vi "c Spark Get Parameter Type.vi"(8 "error in (no error)":errorcluster, 10 "paramID":T1 items=["   c_Spark_kCANID "=0, "    c_Spark_kInputMode "=1, "    c_Spark_kMotorType "=2, "    c_Spark_kCommutationAdvance "=3, "    c_Spark_kControlType "=5, "    c_Spark_kIdleMode "=6, "    c_Spark_kInputDeadband "=7, "    c_Spark_kClosedLoopControlSensor "=9, "    c_Spark_kPolePairs "=10, "    c_Spark_kCurrentChop "=11, "    c_Spark_kCurrentChopCycles "=12, "    c_Spark_kP_0 "=13, "    c_Spark_kI_0 "=14, "    c_Spark_kD_0 "=15, "    c_Spark_kV_0 "=16, "    c_Spark_kIZone_0 "=17, "    c_Spark_kDFilter_0 "=18, "    c_Spark_kOutputMin_0 "=19, "    c_Spark_kOutputMax_0 "=20, "    c_Spark_kP_1 "=21, "    c_Spark_kI_1 "=22, "    c_Spark_kD_1 "=23, "    c_Spark_kV_1 "=24, "    c_Spark_kIZone_1 "=25, "    c_Spark_kDFilter_1 "=26, "    c_Spark_kOutputMin_1 "=27, "    c_Spark_kOutputMax_1 "=28, "    c_Spark_kP_2 "=29, "    c_Spark_kI_2 "=30, "    c_Spark_kD_2 "=31, "    c_Spark_kV_2 "=32, "    c_Spark_kIZone_2 "=33, "    c_Spark_kDFilter_2 "=34, "    c_Spark_kOutputMin_2 "=35, "    c_Spark_kOutputMax_2 "=36, "    c_Spark_kP_3 "=37, "    c_Spark_kI_3 "=38, "    c_Spark_kD_3 "=39, "    c_Spark_kV_3 "=40, "    c_Spark_kIZone_3 "=41, "    c_Spark_kDFilter_3 "=42, "    c_Spark_kOutputMin_3 "=43, "    c_Spark_kOutputMax_3 "=44, "    c_Spark_kInverted "=45, "    c_Spark_kLimitSwitchFwdPolarity "=50, "    c_Spark_kLimitSwitchRevPolarity "=51, "    c_Spark_kHardLimitFwdEn "=52, "    c_Spark_kHardLimitRevEn "=53, "    c_Spark_kSoftLimitFwdEn "=54, "    c_Spark_kSoftLimitRevEn "=55, "    c_Spark_kOpenLoopRampRate "=56, "    c_Spark_kLegacyFollowerID "=57, "    c_Spark_kLegacyFollowerConfig "=58, "    c_Spark_kSmartCurrentStallLimit "=59, "    c_Spark_kSmartCurrentFreeLimit "=60, "    c_Spark_kSmartCurrentConfig "=61, "    c_Spark_kSmartCurrentReserved "=62, "    c_Spark_kMotorKv "=63, "    c_Spark_kEncoderCountsPerRev "=69, "    c_Spark_kEncoderAverageDepth "=70, "    c_Spark_kEncoderSampleDelta "=71, "    c_Spark_kEncoderInverted "=72, "    c_Spark_kVoltageCompensationMode "=74, "    c_Spark_kCompensatedNominalVoltage "=75, "    c_Spark_kIMaxAccum_0 "=96, "    c_Spark_kAllowedClosedLoopError_0 "=97, "    c_Spark_kIMaxAccum_1 "=100, "    c_Spark_kAllowedClosedLoopError_1 "=101, "    c_Spark_kIMaxAccum_2 "=104, "    c_Spark_kAllowedClosedLoopError_2 "=105, "    c_Spark_kIMaxAccum_3 "=108, "    c_Spark_kAllowedClosedLoopError_3 "=109, "    c_Spark_kClosedLoopRampRate "=114, "    c_Spark_kSoftLimitForward "=115, "    c_Spark_kSoftLimitReverse "=116, "    c_Spark_kAnalogAverageDepth "=121, "    c_Spark_kAnalogSensorMode "=122, "    c_Spark_kAnalogInverted "=123, "    c_Spark_kAnalogSampleDelta "=124, "    c_Spark_kCompatibilityPortConfig "=127, "    c_Spark_kAltEncoderCountsPerRev "=128, "    c_Spark_kAltEncoderAverageDepth "=129, "    c_Spark_kAltEncoderSampleDelta "=130, "    c_Spark_kAltEncoderInverted "=131, "    c_Spark_kNumParameters "=138, "    c_Spark_kDutyCycleInverted "=141, "    c_Spark_kDutyCycleAverageDepth "=143, "    c_Spark_kDutyCycleOffsetLegacy "=145, "    c_Spark_kDutyCycleRangeOffset "=146, "    c_Spark_kPositionPIDWrapEnable "=149, "    c_Spark_kDutyCycleSensorPrescaler "=153, "    c_Spark_kDutyCycleOffset "=154, "    c_Spark_kProductId "=155, "    c_Spark_kDeviceMajorVersion "=156, "    c_Spark_kDeviceMinorVersion "=157, "    c_Spark_kStatus0Period "=158, "    c_Spark_kStatus1Period "=159, "    c_Spark_kStatus2Period "=160, "    c_Spark_kStatus3Period "=161, "    c_Spark_kStatus4Period "=162, "    c_Spark_kStatus5Period "=163, "    c_Spark_kStatus6Period "=164, "    c_Spark_kStatus7Period "=165, "    c_Spark_kMAXMotionCruiseVelocity_0 "=166, "    c_Spark_kMAXMotionMaxAccel_0 "=167, "    c_Spark_kMAXMotionMaxJerk_0 "=168, "    c_Spark_kMAXMotionAllowedProfileError_0 "=169, "    c_Spark_kMAXMotionPositionMode_0 "=170, "    c_Spark_kMAXMotionCruiseVelocity_1 "=171, "    c_Spark_kMAXMotionMaxAccel_1 "=172, "    c_Spark_kMAXMotionMaxJerk_1 "=173, "    c_Spark_kMAXMotionAllowedProfileError_1 "=174, "    c_Spark_kMAXMotionPositionMode_1 "=175, "    c_Spark_kMAXMotionCruiseVelocity_2 "=176, "    c_Spark_kMAXMotionMaxAccel_2 "=177, "    c_Spark_kMAXMotionMaxJerk_2 "=178, "    c_Spark_kMAXMotionAllowedProfileError_2 "=179, "    c_Spark_kMAXMotionPositionMode_2 "=180, "    c_Spark_kMAXMotionCruiseVelocity_3 "=181, "    c_Spark_kMAXMotionMaxAccel_3 "=182, "    c_Spark_kMAXMotionMaxJerk_3 "=183, "    c_Spark_kMAXMotionAllowedProfileError_3 "=184, "    c_Spark_kMAXMotionPositionMode_3 "=185, "    c_Spark_kForceEnableStatus_0 "=186, "    c_Spark_kForceEnableStatus_1 "=187, "    c_Spark_kForceEnableStatus_2 "=188, "    c_Spark_kForceEnableStatus_3 "=189, "    c_Spark_kForceEnableStatus_4 "=190, "    c_Spark_kForceEnableStatus_5 "=191, "    c_Spark_kForceEnableStatus_6 "=192, "    c_Spark_kForceEnableStatus_7 "=193, "    c_Spark_kFollowerModeLeaderId "=194, "    c_Spark_kFollowerModeIsInverted "=195, "    c_Spark_kDutyCycleEncoderStartPulseUs "=196, "    c_Spark_kDutyCycleEncoderEndPulseUs "=197, "    c_Spark_kParamTableVersion "=198, "    c_Spark_kStatus8Period "=199, "    c_Spark_kForceEnableStatus_8 "=200, "    c_Spark_kLimitSwitchPositionSensor "=201, "    c_Spark_kLimitSwitchFwdPosition "=202, "    c_Spark_kLimitSwitchRevPosition "=203, "    c_Spark_kS_0 "=204, "    c_Spark_kA_0 "=205, "    c_Spark_kG_0 "=206, "    c_Spark_kCos_0 "=207, "    c_Spark_kCosRatio_0 "=208, "    c_Spark_kS_1 "=209, "    c_Spark_kA_1 "=210, "    c_Spark_kG_1 "=211, "    c_Spark_kCos_1 "=212, "    c_Spark_kCosRatio_1 "=213, "    c_Spark_kS_2 "=214, "    c_Spark_kA_2 "=215, "    c_Spark_kG_2 "=216, "    c_Spark_kCos_2 "=217, "    c_Spark_kCosRatio_2 "=218, "    c_Spark_kS_3 "=219, "    c_Spark_kA_3 "=220, "    c_Spark_kG_3 "=221, "    c_Spark_kCos_3 "=222, "    c_Spark_kCosRatio_3 "=223, "    c_Spark_kStatus9Period "=224, "    c_Spark_kForceEnableStatus_9 "=225, "    c_Spark_kDetachedEncoderDeviceID "=226]) -> (0 "error out":errorcluster, 2 "type":T2(ring))   [LabVIEW 2023, in "REVLibDriver.lvlib"]
doc: "_Spark_GetParameterType"
uses:
  REVLibDriver.lvlib
  REVLibDriver.dll
  Custom Controls/c_Spark_ConfigParameter.ctl
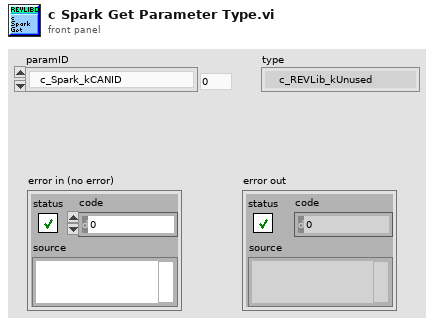
[diagram p1: front panel]
types:
  T1 = typedef "REVLibDriver.lvlib/c_Spark_ConfigParameter.ctl" = u16
  T2 = enum16{"    c_REVLib_kUnused", "    c_REVLib_kInt32", "    c_REVLib_kUint32", "    c_REVLib_kFloat32", "    c_REVLib_kBool"}
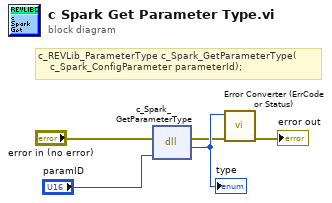
[diagram p0: block diagram]
diagram:
  # "c_REVLib_ParameterType c_Spark_GetParameterType(\n    c_Spark_ConfigParameter parameterId);"
  n1 = dll-call lib="REVLibDriver.*" fn="c_Spark_GetParameterType" ("REVLibDriver:c_Spark_GetParameterBool")(error in="error in (no error)", "paramId"="paramID") -> (error out=w2:errorcluster, "return type"=w5:u32)  [unwired: 3 in, 1 out]
  "type" <- w5
  n2 = call "Error Converter (ErrCode or Status).vi"("error in (no error)"=w2, "error code"=w5) -> ("error out"=→"error out":errorcluster)  [unwired: 9 in]
